vi "Save File DOE Configuration.vi"(5 "Add/Remove Enum":T1(ring)=enum."Update", 7 "Latest String Search":string[](array[string])=["TR Number:", "T0007456"], 8 "error in (no error)":errorcluster, 10 "File Save Configuration Data Path":path=path "C:/GE/Washer DOE/WasherDOEConfig.csv", 11 "Button Number":i32=16) -> (0 "error out":errorcluster, 2 "Updated List":string[](array[string]), 3 "Full Data Output":string[][](array[string])=[["Cycle Selection", "File Paths", "Laurel Meter IP (Cold/Hot)", "Agilent IP", "APLUS IP", "File Search", "ITHX Humidity Sensor IP Address", "Scale IP Address", "Agilent Channels (Analog)", "Agilent Channels (Temperature TC)", "", "Wash Temperature", "Rinse Temperature", "Load Size", "Model Detail Header", "EOC Commands", "Manufacturer-Dish", "Unit Control-Dish", "Test Type:", "Cycle Mode-Dish", "Inlet Temperature-Dish", "Detergent-Dish", "Washer Header Detail", "Dishwasher Header Detail", "TC1 Coefficients (A_B_C)", "TC2 Coefficients (A_B_C)", "TC3 Coefficients (A_B_C)", "TC4 Coefficients (A_B_C)", "TC5 Coefficients (A_B_C)", "TC6 Coefficients (A_B_C)", "TC7 Coefficients (A_B_C)", "TR Number:", "Lab ID:", "Station ID:", "Technician:", "Water Pressure (PSI):", "Ambient RH:", "Supply Voltage:", "Frequency:", "Build:", "Hot Water Temperature (Fahrenheit)", "Cold Water Temperature (Fahrenheit)", "Heating Mode"], ["Eco Wash", "C:\\GE\\Washer DOE\\CalibrationDates.txt", "10.0.3.67", "169.254.9.72", "10.0.3.101", "DOE Template", "10.0.3.139", "10.0.3.5", "101", "111", "", "Extra Hot", "Cold", "Max", "TR Number:", "EOC", "GE", "Electronic", "Kitchen", "Auto", "110", "Cascade", "Program Name:", "Manufacturer:", "0", "0", "0", "0", "0", "0", "0", "", "", "Station 1", "Test", "25", "50", "110", "50", "DG", "120", "50", "Heat Pump"], ["Standard Wash", "C:\\GE\\Washer DOE\\DOE Capacity.txt", "10.0.3.66", "", "", "Rev", "", "", "102", "112", "", "Hot", "Hot Rinse", "Min", "Lab ID:", "ShuttingDown", "Electrolux", "Mechanical", "DOE", "Pots & Pans", "120", "Dawn", "Model Family:", "Unit Control:", "0", "0", "0", "0", "0", "0", "0", "", "", "Station 2", "", "30", "60", "115", "60", "DC", "130", "58", "Hybrid"], ["Heavy Wash", "C:\\GE\\Washer DOE", "", "", "", "xltm", "", "", "113", "", "", "Warm 1", "", "Avg", "Test Name:", "", "Mabe", "", "Portable Test", "Quick", "130", "Gain", "Cycle Selection:", "Test Type:", "0", "0", "0", "0", "0", "0", "0", "", "", "Station 3", "", "35", "80", "120", "80", "Pre-Pilot", "135", "68", "Boost"], ["test", "\\\\3.67.38.12\\share\\Test Data\\Washer DOE\\Models", "", "", "", "", "", "", "114", "", "", "Warm 2", "", "Max1*", "Model:", "", "Bosch", "", "", "", "135", "", "Wash Temperature:", "Cycle Mode:", "", "", "", "", "", "", "", "", "", "Station 4", "", "40", "60", "140", "", "Production", "140", "", "Standard"], ["", "D:\\data\\WasherDOE", "", "", "", "", "", "", "115", "", "", "Warm 3", "", "Max2**", "Serial Number:", "", "Whirlpool", "", "", "", "140", "", "Rinse Temperature:", "Inlet Temperature (F):", "", "", "", "", "", "", "", "", "", "Station 5", "", "", "", "", "", "", "", "", "Vacation"], ["", "C:\\GE\\Washer DOE\\DOE_Backup.ini", "", "", "", "", "", "", "116", "", "", "Cold", "", "", "Station ID:", "", "", "", "", "", "", "", "Load Size:", "Detergent:", "", "", "", "", "", "", "", "", "", "Station 6", "", "", "", "", "", "", "", "", ""], ["", "", "", "", "", "", "", "", "", "", "", "Note", "", "", "Engineer:", "", "", "", "", "", "", "", "Hot Water Temperature (Fahrenheit):", "Auto Cup Weight (gm):", "", "", "", "", "", "", "", "", "", "Station 7", "", "", "", "", "", "", "", "", ""], ["", "", "", "", "", "", "", "", "", "", "", "", "", "", "Technician", "", "", "", "", "", "", "", "Cold Water Temperature (Fahrenheit):", "Open Cup Weight (gm):", "", "", "", "", "", "", "", "", "", "Station 8", "", "", "", "", "", "", "", "", ""], ["", "", "", "", "", "", "", "", "", "", "", "", "", "", "Water Pressure:", "", "", "", "", "", "", "", "Capacity (cu.ft)", "", "", "", "", "", "", "", "", "", "", "Station 9", "", "", "", "", "", "", "", "", ""], ["", "", "", "", "", "", "", "", "", "", "", "", "", "", "Ambient RH:", "", "", "", "", "", "", "", "Initial Cloth Weight:", "", "", "", "", "", "", "", "", "", "", "Station 10", "", "", "", "", "", "", "", "", ""], ["", "", "", "", "", "", "", "", "", "", "", "", "", "", "Supply Voltage:", "", "", "", "", "", "", "", "Cloth Lot:", "", "", "", "", "", "", "", "", "", "", "Station 11", "", "", "", "", "", "", "", "", ""], ["", "", "", "", "", "", "", "", "", "", "", "", "", "", "Frequency:", "", "", "", "", "", "", "", "", "", "", "", "", "", "", "", "", "", "", "Station 12", "", "", "", "", "", "", "", "", ""], ["", "", "", "", "", "", "", "", "", "", "", "", "", "", "Build:", "", "", "", "", "", "", "", "", "", "", "", "", "", "", "", "", "", "", "", "", "", "", "", "", "", "", "", ""]])   [LabVIEW 2023, in "File Setup.lvlib"]
uses:
  File Setup.lvlib
  <vilib>/Utility/file.llb/Read Delimited Spreadsheet (string).vi
  <vilib>/Utility/file.llb/Write Delimited Spreadsheet (string).vi
panel:
  in  "Configuration Tab":enum32{"Main", "Default Data", "Configuration"}(tab)=enum."Default Data"
  in  "Calibration Data":string[][](array[string])
  in  "Update":bool
  out "Default Data Output":string[][](array[string])
  out "Coeffficient C":dbl
  out "Coeffficient B":dbl
  out "Coeffficient A":dbl
  in  "Get Coefficients":bool
  in  "TC Inputs":string[][](array[string])=[["Temperature Setpoint", "Sourced TC Temperature (F)", "Measured TC Temperature (F)"], ["1", "", ""], ["2", "", ""], ["3", "", ""]]
  in  "Debug Tab":enum32{"Input", "Output"}(tab)
  in  "Debug":bool=TRUE
  out "States":string[](array[string])=["Macro: Initialize", "Data: Initialize", "Initialize Core Data", "UI: Initialize", "UI: Front Panel State", "Read Current Data"]
  # "Configuration File Update"
  # "Calculate TC Coefficients"
  # "Agilent Syntax\n\nY=Gain*x+Offset = (Gain_Offset_Name)Channel_AG# or (5.23_3.4_TC1)107_1"
  # "Kitchen TC Layout\n\n1) TC Jack 1\n2) TC Jack 2\n3) TC Jack 3\n4) TC Jack 4\n5) TC Jack 5\n6) TC Jack 6\n7) Hot Water TC"
  # "Washer DOE\n\n1) TC1 Cold Water Temp\n2) TC2 Hot Water Temp\n3) N/A\n4) N/A\n5) N/A\n6) N/A\n7) N/A"
  # "Portable Adv Sys\n\n1) TC1 Cold Water Temp\n2) TC2 Hot Water Temp\n3) N/A\n4) N/A\n5) N/A\n6) N/A\n7) N/A"
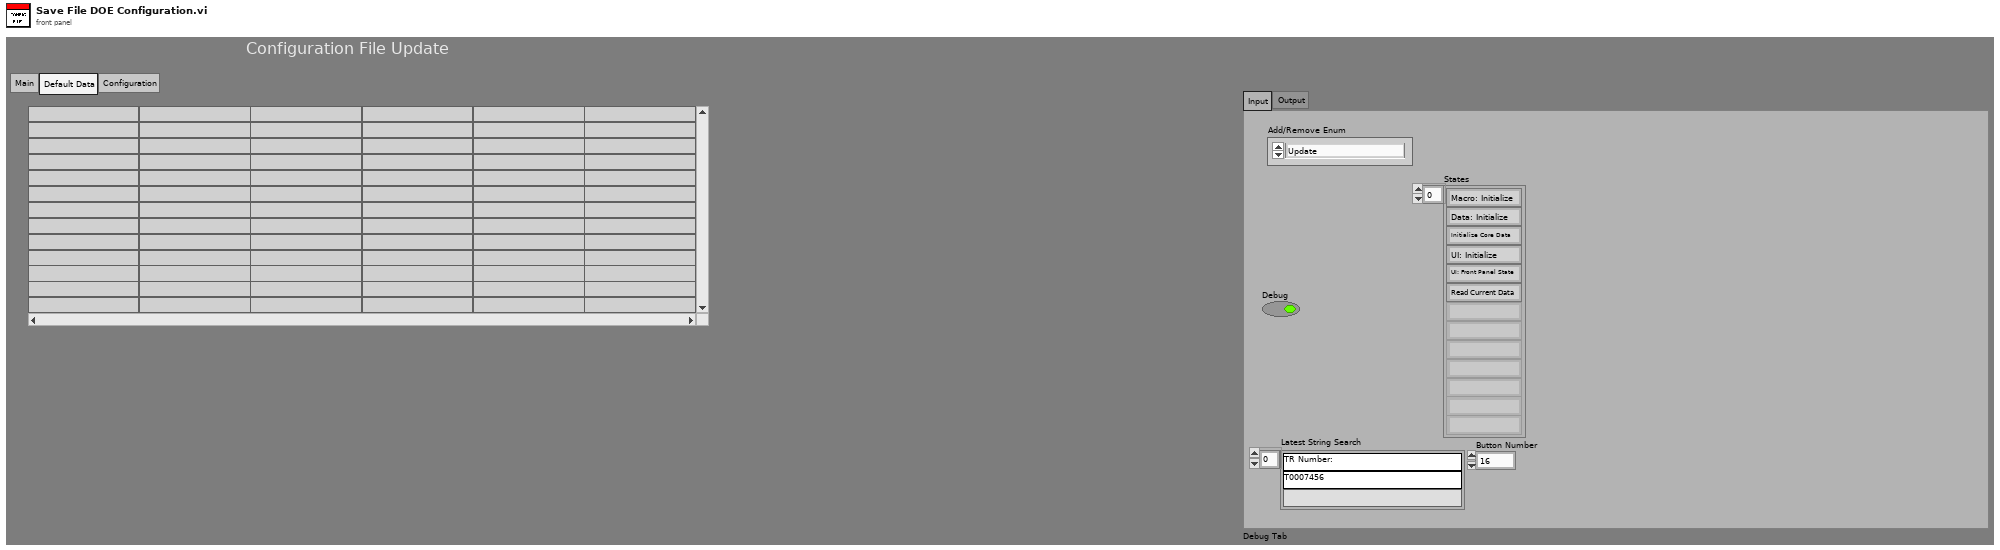
[diagram p1: front panel]
types:
  T1 = enum16{"Load Standard", "Remove", "Add", "Update"}
  T2 = enum32{"invalid app kind", "Development System", "Run Time System", "Student Edition", "Embedded LabVIEW", "Evaluation", "Custom"}
  T3 = enum32{"Invalid", "Standard", "Closed", "Hidden", "Minimized", "Maximized"}
  T4 = cluster{"Core":cluster{"Current VI Reference":refnum<vi>, "Close Panel on Exit?":bool}, "File Save Configuration Data Path":path, "Full Data":string[][], "Button Number":i32, "Latest String Search":string[], "Updated List":string[]}
  T5 = cluster{"Current VI Reference":refnum<vi>, "Close Panel on Exit?":bool}
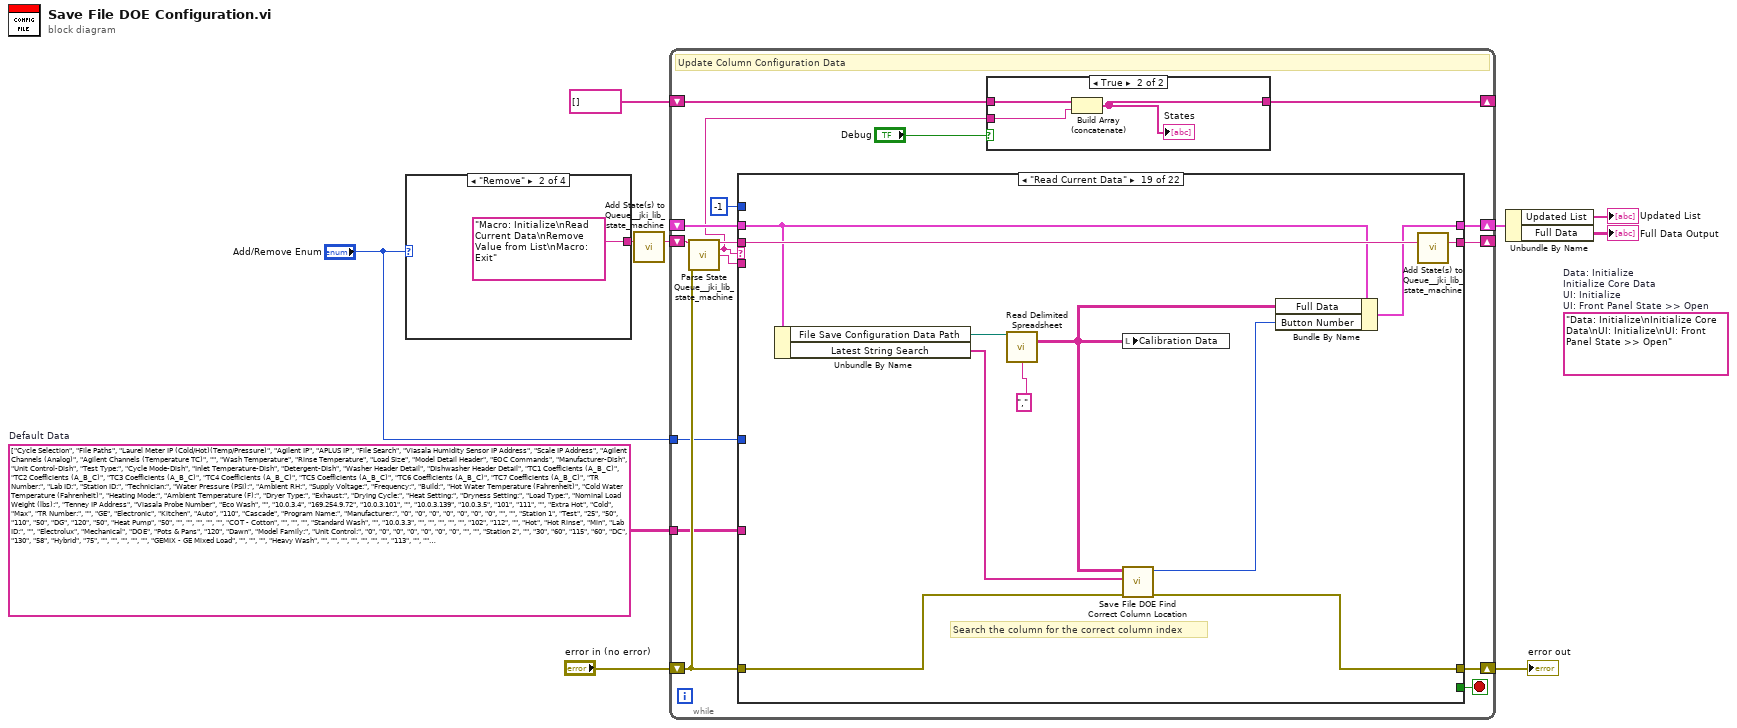
[diagram p0: block diagram]
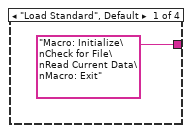
[diagram p2: hidden frame]
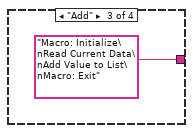
[diagram p3: hidden frame]
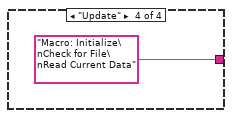
[diagram p4: hidden frame]
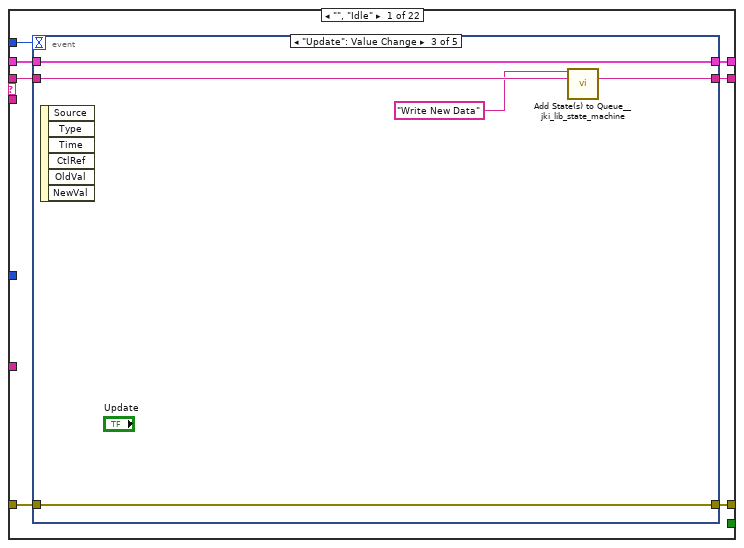
[diagram p6: hidden frame]
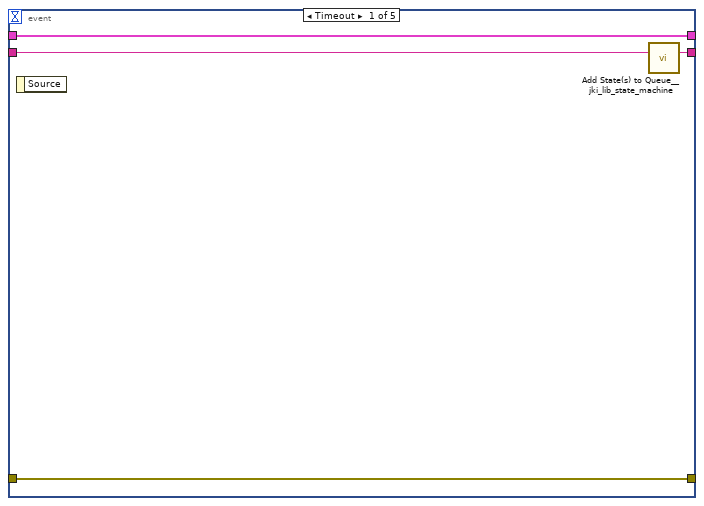
[diagram p7: hidden frame]
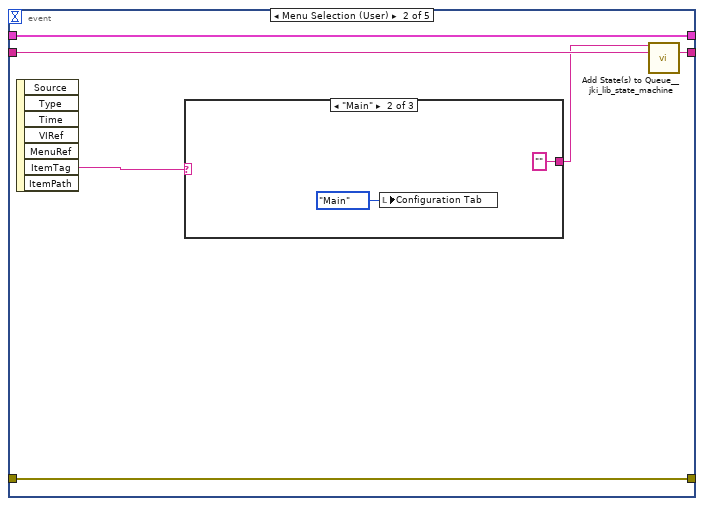
[diagram p8: hidden frame]
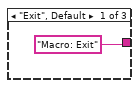
[diagram p9: hidden frame]
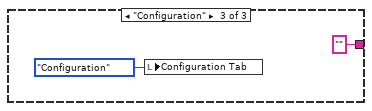
[diagram p10: hidden frame]
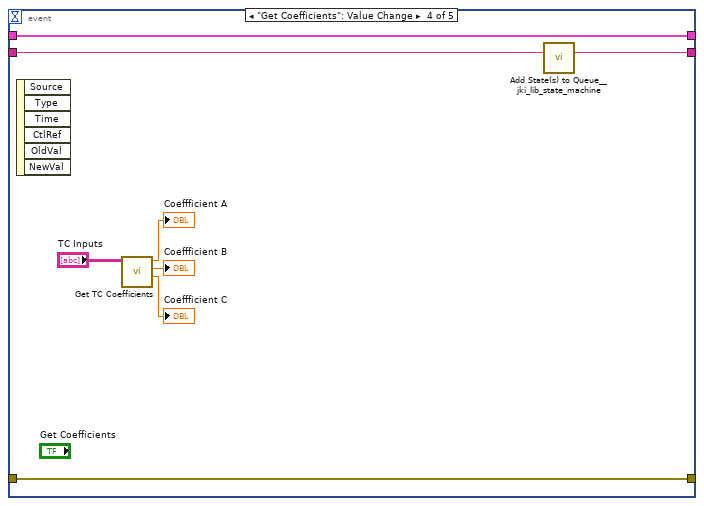
[diagram p11: hidden frame]
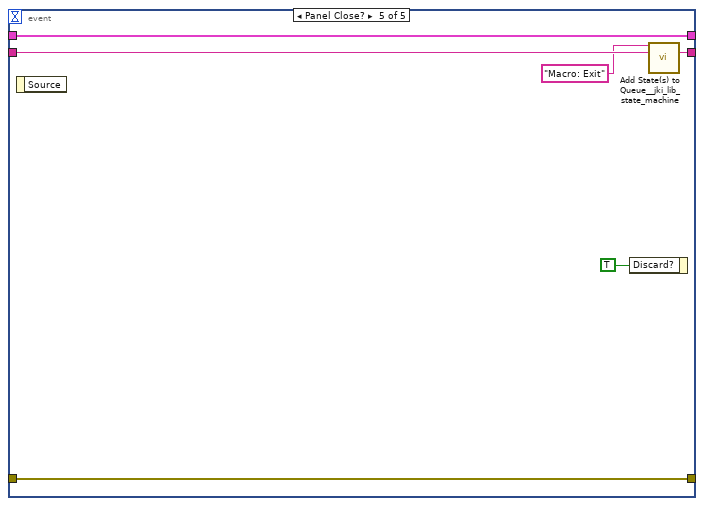
[diagram p12: hidden frame]
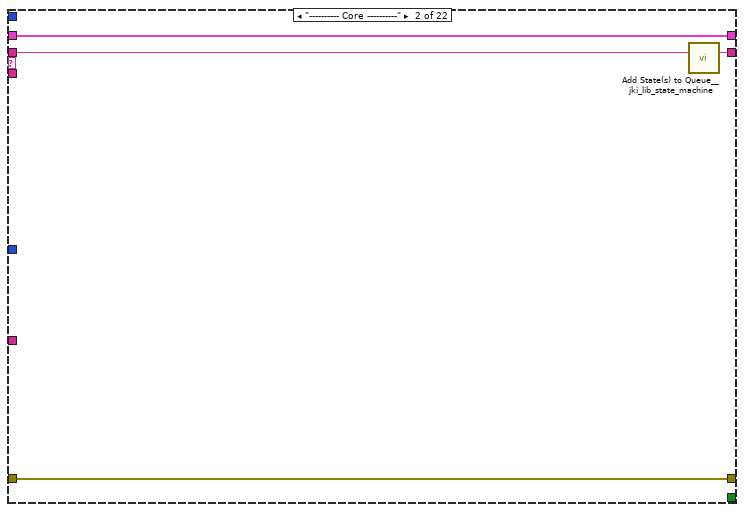
[diagram p13: hidden frame]
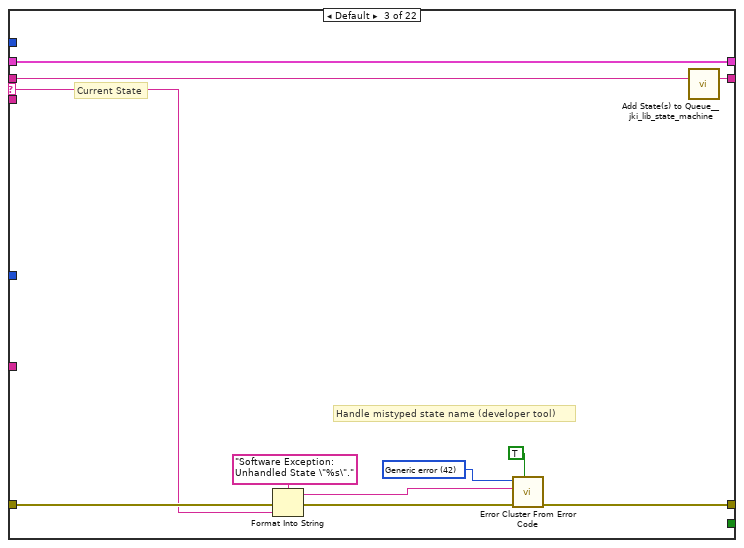
[diagram p14: hidden frame]
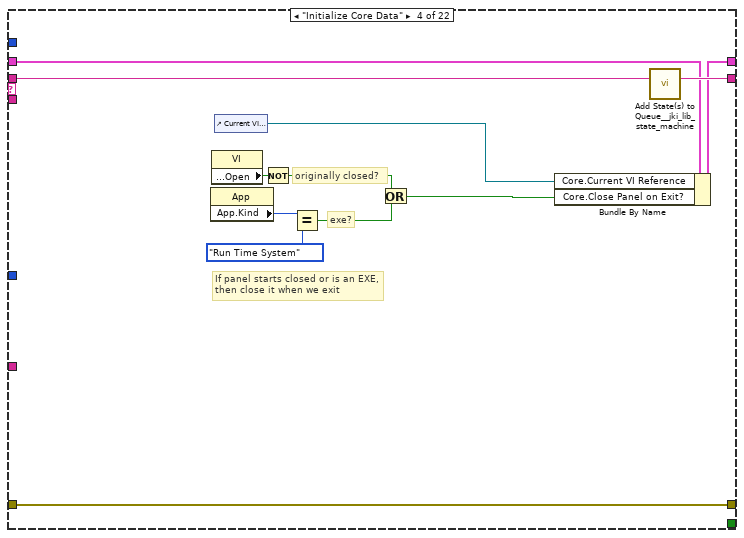
[diagram p15: hidden frame]
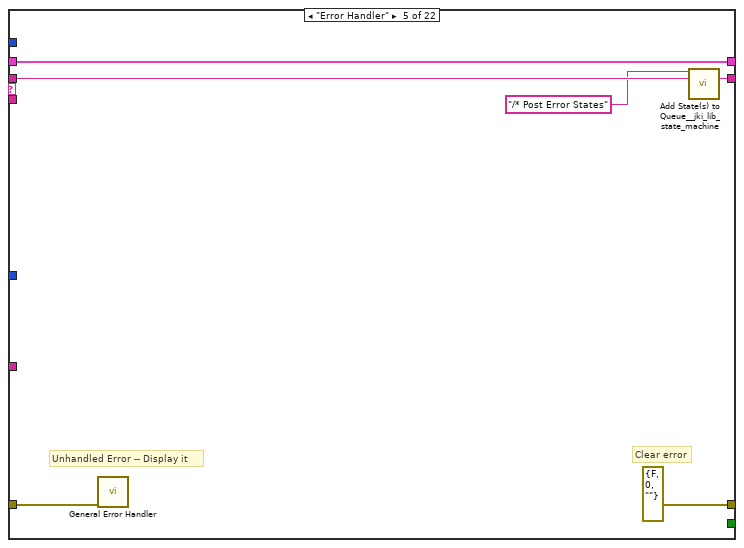
[diagram p16: hidden frame]
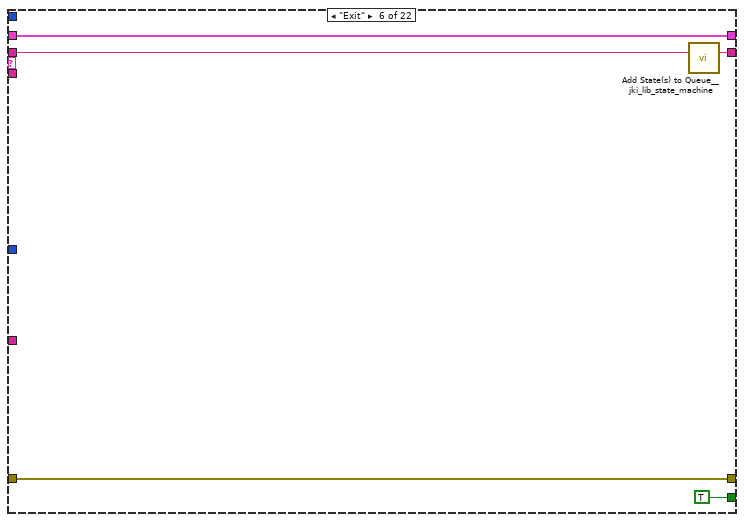
[diagram p17: hidden frame]
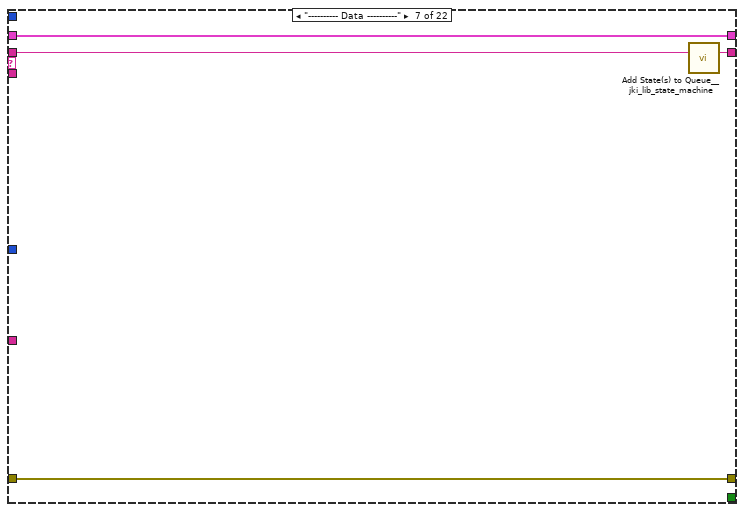
[diagram p18: hidden frame]
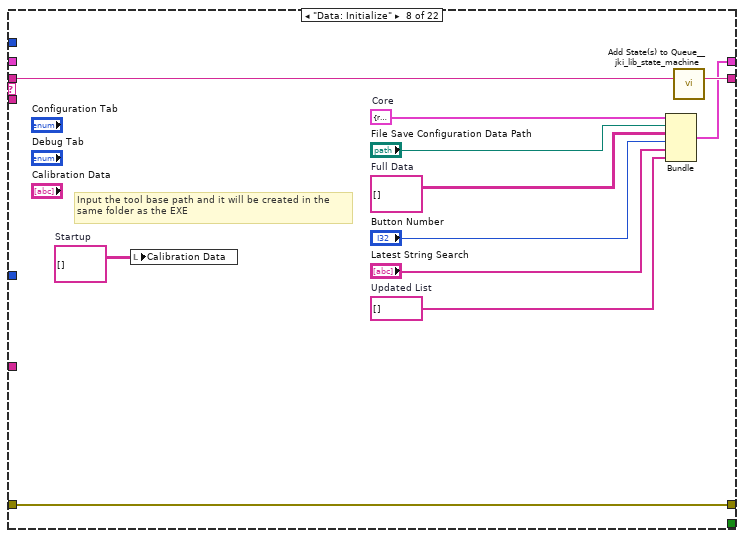
[diagram p19: hidden frame]
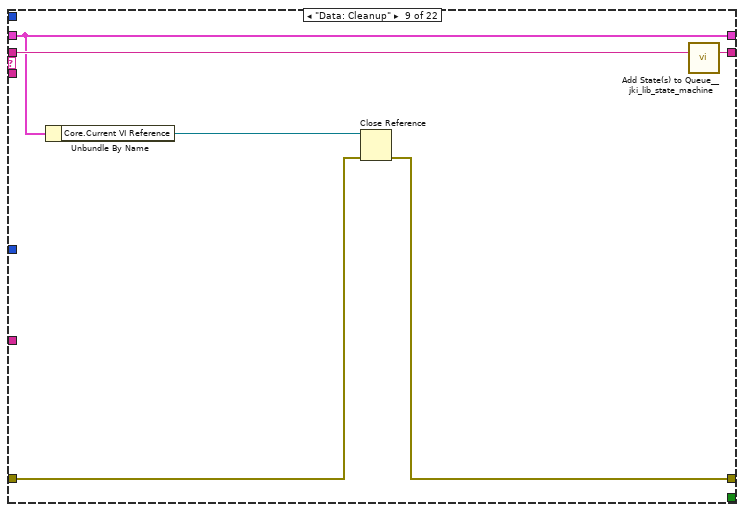
[diagram p20: hidden frame]
diagram:
  (unwired) "Data: Initialize\nInitialize Core Data\nUI: Initialize\nUI: Front Panel State >> Open"  # Data: Initialize Initialize Core Data UI: Initialize UI: Front Panel State >> Open
  w1 = string[][] [["Cycle Selection", "File Paths", "Laurel Meter IP (Cold/Hot)(Temp/Pressure)", "Agilent IP", "APLUS IP", "File Search", "Viasala Humidity Sensor IP Address", "Scale IP Address", "Agilent Channels (Analog)", "Agilent Channels (Temperature TC)", "", "Wash Temperature", "Rinse Temperature", "Load Size", "Model Detail Header", "EOC Commands", "Manufacturer-Dish", "Unit Control-Dish", "Test Type:", "Cycle Mode-Dish", "Inlet Temperature-Dish", "Detergent-Dish", "Washer Header Detail", "Dishwasher Header Detail", "TC1 Coefficients (A_B_C)", "TC2 Coefficients (A_B_C)", "TC3 Coefficients (A_B_C)", "TC4 Coefficients (A_B_C)", "TC5 Coefficients (A_B_C)", "TC6 Coefficients (A_B_C)", "TC7 Coefficients (A_B_C)", "TR Number:", "Lab ID:", "Station ID:", "Technician:", "Water Pressure (PSI):", "Ambient RH:", "Supply Voltage:", "Frequency:", "Build:", "Hot Water Temperature (Fahrenheit)", "Cold Water Temperature (Fahrenheit)", "Heating Mode:", "Ambient Temperature (F):", "Dryer Type:", "Exhaust:", "Drying Cycle:", "Heat Setting:", "Dryness Setting:", "Load Type:", "Nominal Load Weight (lbs):", "Tenney IP Address", "Viasala Probe Number"], ["Eco Wash", "", "10.0.3.4", "169.254.9.72", "10.0.3.101", "", "10.0.3.139", "10.0.3.5", "101", "111", "", "Extra Hot", "Cold", "Max", "TR Number:", "", "GE", "Electronic", "Kitchen", "Auto", "110", "Cascade", "Program Name:", "Manufacturer:", "0", "0", "0", "0", "0", "0", "0", "", "", "Station 1", "Test", "25", "50", "110", "50", "DG", "120", "50", "Heat Pump", "50", "", "", "", "", "", "COT - Cotton", "", "", ""], ["Standard Wash", "", "10.0.3.3", "", "", "", "", "", "102", "112", "", "Hot", "Hot Rinse", "Min", "Lab ID:", "", "Electrolux", "Mechanical", "DOE", "Pots & Pans", "120", "Dawn", "Model Family:", "Unit Control:", "0", "0", "0", "0", "0", "0", "0", "", "", "Station 2", "", "30", "60", "115", "60", "DC", "130", "58", "Hybrid", "75", "", "", "", "", "", "GEMIX - GE Mixed Load", "", "", ""], ["Heavy Wash", "", "", "", "", "", "", "", "113", "", "", "Warm 1", "", "Avg", "Test Name:", "", "Mabe", "", "Portable Test", "Quick", "130", "Gain", "Cycle Selection:", "Test Type:", "0", "0", "0", "0", "0", "0", "0", "", "", "Station 3", "", "35", "80", "120", "80", "Pre-Pilot", "135", "68", "Boost", "90", "", "", "", "", "", "GEEZ - GE Easy Care", "", "", ""], ["test", "", "", "", "", "", "", "", "", "", "", "Warm 2", "", "Max1*", "Model:", "", "Bosch", "", "", "", "135", "", "Wash Temperature:", "Cycle Mode:", "", "", "", "", "", "", "", "", "", "Station 4", "", "40", "60", "140", "", "Production", "140", "", "Standard", "", "", "", "", "", "", "GEDEL - Ge Delicate Load (CU)", "", "", ""], ["", "C:\\data", "", "", "", "", "", "", "", "", "", "Warm 3", "", "Max2**", "Serial Number:", "", "Whirlpool", "", "", "", "140", "", "Rinse Temperature:", "Inlet Temperature (F):", "", "", "", "", "", "", "", "", "", "Station 5", "", "", "", "", "", "", "", "", "Vacation", "", "", "", "", "", "", "CU - CU Load", "", "", ""], ["", "C:\\GE\\Washer DOE\\DOE_Backup.ini", "", "", "", "", "", "", "", "", "", "Cold", "", "", "Station ID:", "", "", "", "", "", "", "", "Load Size:", "Detergent:", "", "", "", "", "", "", "", "", "", "Station 6", "", "", "", "", "", "", "", "", "", "", "", "", "", "", "", "DOE", "", "", ""], ["", "", "", "", "", "", "", "", "", "", "", "Note", "", "", "Engineer:", "", "", "", "", "", "", "", "Hot Water Temperature (Fahrenheit):", "Auto Cup Weight (gm):", "", "", "", "", "", "", "", "", "", "Station 7", "", "", "", "", "", "", "", "", "", "", "", "", "", "", "", "UL", "", "", ""], ["", "", "", "", "", "", "", "", "", "", "", "", "", "", "Technician", "", "", "", "", "", "", "", "Cold Water Temperature (Fahrenheit):", "Open Cup Weight (gm):", "", "", "", "", "", "", "", "", "", "Station 8", "", "", "", "", "", "", "", "", "", "", "", "", "", "", "", "AHAM", "", "", ""], ["", "", "", "", "", "", "", "", "", "", "", "", "", "", "Water Pressure:", "", "", "", "", "", "", "", "Capacity (cu.ft)", "", "", "", "", "", "", "", "", "", "", "Station 9", "", "", "", "", "", "", "", "", "", "", "", "", "", "", "", "GEACT", "", "", ""], ["", "", "", "", "", "", "", "", "", "", "", "", "", "", "Ambient RH:", "", "", "", "", "", "", "", "Initial Cloth Weight:", "", "", "", "", "", "", "", "", "", "", "Station 10", "", "", "", "", "", "", "", "", "", "", "", "", "", "", "", "", "", "", ""], ["", "", "", "", "", "", "", "", "", "", "", "", "", "", "Supply Voltage:", "", "", "", "", "", "", "", "Cloth Lot:", "", "", "", "", "", "", "", "", "", "", "Station 11", "", "", "", "", "", "", "", "", "", "", "", "", "", "", "", "", "", "", ""], ["", "", "", "", "", "", "", "", "", "", "", "", "", "", "Frequency:", "", "", "", "", "", "", "", "", "", "", "", "", "", "", "", "", "", "", "Station 12", "", "", "", "", "", "", "", "", "", "", "", "", "", "", "", "", "", "", ""], ["", "", "", "", "", "", "", "", "", "", "", "", "", "", "Build:", "", "", "", "", "", "", "", "", "", "", "", "", "", "", "", "", "", "", "", "", "", "", "", "", "", "", "", "", "", "", "", "", "", "", "", "", "", ""]]  # Default Data
  n1 = case shown="\"Remove\"" "Add/Remove Enum" {
    tunnel: ["Macro: Initialize\nCheck for File\nRead Current Data\nMacro: Exit" "Macro: Initialize\nRead Current Data\nRemove Value from List\nMacro: Exit" "Macro: Initialize\nRead Current Data\nAdd Value to List\nMacro: Exit" "Macro: Initialize\nCheck for File\nRead Current Data"] -> w9
    frame "Load Standard", Default {
    }
    frame "Remove" {
    }
    frame "Add" {
    }
    frame "Update" {
    }
  }
  n2 = call <vilib>:"Add State(s) to Queue__jki_lib_state_machine.vi"("State(s) in (\"\")"=w9) -> ("States Out"=w10:string)  [unwired: 14 in]
  n3 = while "Update Column Configuration Data" {
    shift-right: [w24] -> w5
    shift-left: _ -> [w23]
    shift-right: [w27] -> w8
    shift-left: "error in (no error)" -> [w21]
    shift-right: [w26] -> _
    shift-left: w10 -> [w28]
    tunnel: "Add/Remove Enum" -> [w20]
    shift-right: [w17] -> _
    shift-left: string[] [] -> [w18]
    tunnel: w1 -> [w15]
    stop <- w25 stop-if-true
    # "Update Column Configuration Data"
    n4 = call <vilib>:"Parse State Queue__jki_lib_state_machine.vi"("State Queue"=w28, "Error In (no error)"=w21) -> ("Remaining States"=w30:string, "Current State"=w19:string, "Arguments"=w29:string)  [unwired: 11 in]
    n5 = case shown="\"Read Current Data\"" w19 {
      selector: w19 -> [_ _ w80 _ _ _ _ _ _ _ _ _ _ _ _ _ _ _ _ _ _ _]
      tunnel: w30 -> [w41 w79 w84 w102 w108 w113 w117 w128 w134 w138 w142 w148 w159 w185 w190 w200 w204 w213 w229 w238 w257 w276]
      tunnel: w29 -> [_ _ _ _ _ _ _ _ _ _ _ w143 w153 _ _ _ _ _ _ _ _ _]
      tunnel: w23 -> [w39 w76 w82 w93 w105 w111 w114 _ w129 w135 w139 w146 w155 w182 w187 w197 w201 w211 w225 w234 w252 w272]
      tunnel: [w38 w77 w86 w99 errorcluster {"status"=FALSE, "code"=0, "source"=""} ("error out") w110 w115 w125 w130 w136 w140 w144 w156 w183 w188 w198 w202 w206 w221 w236 w255 w274] -> w27
      tunnel: w21 -> [w37 w77 w85 w99 w104 w110 w115 w125 w131 w136 w140 w145 w157 w183 w188 w198 w202 w209 w222 w236 w255 w274]
      tunnel: [w40 w78 w83 w101 w107 w112 w116 w127 w133 w137 w141 w147 w158 w184 w189 w199 w203 w212 w228 w237 w256 w275] -> w26
      tunnel: [_ _ _ _ _ TRUE _ _ _ _ _ _ _ _ _ _ _ _ _ _ _ _] -> w25
      tunnel: [w36 w76 w82 w100 w105 w111 w114 w126 w129 w135 w139 w146 w155 w182 w187 w197 w201 w211 w224 w234 w251 w271] -> w24
      tunnel: -1 ("Timeout") -> [w35 _ _ _ _ _ _ _ _ _ _ _ _ _ _ _ _ _ _ _ _ _]
      tunnel: w20 -> [_ _ _ _ _ _ _ _ _ _ _ _ _ _ _ _ _ _ _ w232 _ _]
      tunnel: w15 -> [_ _ _ _ _ _ _ _ _ _ _ _ _ _ _ _ _ w205 _ _ _ _]
      frame "", "Idle" {
        n6 = event shown="[2] \"Update\": Value Change" {
          selector: _ -> [_ _ _ _ _]
          dyn-events: _ -> [_ _ _ _ _]
          timeout: w35 -> [_ _ _ _ _]
          tunnel: w41 -> [w45 w51 w59 w67 w75]
          tunnel: [w44 w50 w58 w66 w74] -> w40
          tunnel: w39 -> [w42 w48 w61 w69 w72]
          tunnel: [w43 w49 w60 w68 w73] -> w38
          tunnel: w37 -> [w43 w49 w60 w68 w73]
          tunnel: [w42 w48 w61 w69 w72] -> w36
          event Timeout {
            n7 = event-data() -> ()  [unwired: 1 in, 1 out]
            n8 = call <vilib>:"Add State(s) to Queue__jki_lib_state_machine.vi"("State(s) in (\"\")"=w45) -> ("States Out"=w44:string)  [unwired: 14 in]
          }
          event Menu Selection (User) {
            n9 = event-data() -> ("ItemTag"=w47:string)  [unwired: 1 in, 6 out]
            n10 = case shown="\"Main\"" w47 {
              tunnel: ["Macro: Exit" "" ""] -> w46
              frame "Exit", Default {
              }
              frame "Main" {
                n11 = local write "Configuration Tab"(enum32{"Main", "Default Data", "Configuration"}."Main" ("Configuration Tab")) -> ()
              }
              frame "Configuration" {
                n12 = local write "Configuration Tab"(enum32{"Main", "Default Data", "Configuration"}."Configuration" ("Configuration Tab")) -> ()
              }
            }
            n13 = call <vilib>:"Add State(s) to Queue__jki_lib_state_machine.vi"("State(s) in Front (\"\")"=w46, "State(s) in (\"\")"=w51) -> ("States Out"=w50:string)  [unwired: 13 in]
          }
          event "Update": Value Change {
            n14 = event-data() -> ()  [unwired: 1 in, 6 out]
            n15 = call <vilib>:"Add State(s) to Queue__jki_lib_state_machine.vi"("State(s) in Front (\"\")"="Write New Data" ("State(s) in Front (\"\")"), "State(s) in (\"\")"=w59) -> ("States Out"=w58:string)  [unwired: 13 in]
          }
          event "Get Coefficients": Value Change {
            n16 = event-data() -> ()  [unwired: 1 in, 6 out]
            n17 = call "Get TC Coefficients.vi"("TC Inputs"="TC Inputs") -> ("C"=→"Coeffficient C":dbl, "B"=→"Coeffficient B":dbl, "A"=→"Coeffficient A":dbl)  [unwired: 8 in]
            n18 = call <vilib>:"Add State(s) to Queue__jki_lib_state_machine.vi"("State(s) in (\"\")"=w67) -> ("States Out"=w66:string)  [unwired: 14 in]
          }
          event Panel Close? {
            n19 = event-data() -> ()  [unwired: 1 in, 1 out]
            n20 = event-data("Discard?"=TRUE) -> ()  [unwired: 1 in, 1 out]
            n21 = call <vilib>:"Add State(s) to Queue__jki_lib_state_machine.vi"("State(s) in Front (\"\")"="Macro: Exit", "State(s) in (\"\")"=w75) -> ("States Out"=w74:string)  [unwired: 13 in]
          }
        }
      }
      frame "---------- Core ----------" {
        n22 = call <vilib>:"Add State(s) to Queue__jki_lib_state_machine.vi"("State(s) in (\"\")"=w79) -> ("States Out"=w78:string)  [unwired: 14 in]
      }
      frame Default {
        w89 = 42 items=["No error", "Argument error", "Memory is full", "Out of zone", "End of file", "File already open", "Generic file I/O error", "File not found", "File permission error", "Disk is full", "Duplicate path", "Too many files open", "System feature not enabled", "Resource file not found", "Cannot add resource", "Resource not found", "Image not found", "Image memory error", "Pen does not exist", "Config type invalid", "Config token not found", "Config parse error", "Config memory error", "Bad external code format", "Bad external code offset", "External code not present", "Null window", "Destroy window error", "Null menu", "Print aborted", "Bad print record", "Print driver error", "Windows error during printing", "Memory error during printing", "Print dialog error", "Generic print error", "Invalid device refnum", "Device not found", "Device parameter error", "Device unit error", "Cannot open device", "Device call aborted", "Generic error", "Cancelled by user", "Object ID too low", "Object ID too high", "Object not in heap", "Unknown heap", "Unknown object (invalid DefProc)", "Unknown object (DefProc not in table)", "Message out of range", "Invalid (null) method", "Unknown message", "Manager call not supported", "Bad address", "Network operation in progress", "Network operation timed out", "Connection is busy", "Network attribute not supported", "Network error", "Address in use", "System out of memory", "Connection aborted", "Connection refused", "Not connected", "Already connected", "Connection closed", "Initialization error (interapplication manager)", "Bad occurrence", "Wait on unbound occurrence handler", "Occurrence queue overflow", "Datalog type conflict", "Unused", "Unrecognized type (interapplication manager)", "Memory corrupt", "Failed to make temporary DLL", "Old CIN version", "Drag socket not found", "Failed to load drop-object", "Failed to register OLE object", "Failed to release OLE object", "Format specifier type mismatch", "Unknown format specifier", "Too few format specifiers", "Too many format specifiers", "Scan failed", "Newer CIN version", "Error converting to variant", "Runtime menu error", "Password tampered", "Variant attribute not found", "Incompatible variant data type", "Event data is not available", "Event Store is not present", "Occurrence is not found", "Event Queue is not created", "Event info is not available", "Refnum passed is NULL", "Error retrieving Class GUID", "Error retrieving CoClass GUID", "Error retrieving TypeLib GUID.", "Bad built application magic bytes.", "Specific driver is different from the specific driver associated with the Logical Name.", "There is no session opened to the class driver.", "Max Error", "MAX - Error with config objects", "MAX - Error loading configuration", "MAX - Group not supported"]
        # "Current State"
        # "Handle mistyped state name (developer tool)"
        n23 = Format Into String(format string="Software Exception: Unhandled State \"%s\"." ("message"), error in=w85, w80) -> (resulting string=w88:string, error out=w87:errorcluster)  [unwired: 1 in]
        n24 = call <vilib>:"Error Cluster From Error Code.vi"("show call chain? (False)"=TRUE, "error in (no error)"=w87, "error message (\"\")"=w88, "error code (0)"=w89) -> ("error out"=w86:errorcluster)  [unwired: 5 in]
        n25 = call <vilib>:"Add State(s) to Queue__jki_lib_state_machine.vi"("State(s) in (\"\")"=w84) -> ("States Out"=w83:string)  [unwired: 14 in]
      }
      frame "Initialize Core Data" {
        # "originally closed?"
        # "exe?"
        # "If panel starts closed or is an EXE, then close it when we exit"
        n26 = property class="App"() -> ("App.Kind"=w97:T2)  [unwired: 2 in, 2 out]
        n27 = property class="VI"() -> ("Front Panel.Open"=w98:bool)  [unwired: 2 in, 2 out]
        n28 = control-ref of="Current VI Reference"() -> (w91:refnum<vi>)
        n29 = Not(x=w98) -> (.not. x?=w95:bool)
        n30 = Equal?(x=w97, y=T2."Run Time System" ("Application:Kind")) -> (x = y?=w94:bool)
        n31 = Or(x=w95, y=w94) -> (x .or. y?=w92:bool)
        n32 = Bundle By Name(cluster=w93, "Core.Current VI Reference"=w91, "Core.Close Panel on Exit?"=w92) -> (w100:T4)
        n33 = call <vilib>:"Add State(s) to Queue__jki_lib_state_machine.vi"("State(s) in (\"\")"=w102) -> ("States Out"=w101:string)  [unwired: 14 in]
      }
      frame "Error Handler" {
        # "Unhandled Error -- Display it"
        # "Clear error"
        n34 = call <vilib>:"General Error Handler.vi"("error in (no error)"=w104) -> ()  [unwired: 10 in, 5 out]
        n35 = call <vilib>:"Add State(s) to Queue__jki_lib_state_machine.vi"("State(s) in Front (\"\")"="/* Post Error States", "State(s) in (\"\")"=w108) -> ("States Out"=w107:string)  [unwired: 13 in]
      }
      frame "Exit" {
        n36 = call <vilib>:"Add State(s) to Queue__jki_lib_state_machine.vi"("State(s) in (\"\")"=w113) -> ("States Out"=w112:string)  [unwired: 14 in]
      }
      frame "---------- Data ----------" {
        n37 = call <vilib>:"Add State(s) to Queue__jki_lib_state_machine.vi"("State(s) in (\"\")"=w117) -> ("States Out"=w116:string)  [unwired: 14 in]
      }
      frame "Data: Initialize" {
        w119 = string[][] []  # Startup
        w121 = string[] []  # Updated List
        w123 = string[][] []  # Full Data
        w124 = T5 {"Current VI Reference"=refnum, "Close Panel on Exit?"=TRUE}  # Core
        # "Input the tool base path and it will be created in the \nsame folder as the EXE"
        n38 = local write "Calibration Data"(w119) -> ()
        n39 = Bundle("Core"=w124, "File Save Configuration Data Path"="File Save Configuration Data Path", "Full Data"=w123, "Button Number"="Button Number", "Latest String Search"="Latest String Search", "Updated List"=w121) -> (w126:T4)  [unwired: 1 in]
        n40 = call <vilib>:"Add State(s) to Queue__jki_lib_state_machine.vi"("State(s) in (\"\")"=w128) -> ("States Out"=w127:string)  [unwired: 14 in]
      }
      frame "Data: Cleanup" {
        n41 = Unbundle By Name(w129) -> ("Core.Current VI Reference"=w132:refnum<vi>)
        n42 = Close Reference(reference=w132, error in (no error)=w131) -> (error out=w130:errorcluster)
        n43 = call <vilib>:"Add State(s) to Queue__jki_lib_state_machine.vi"("State(s) in (\"\")"=w134) -> ("States Out"=w133:string)  [unwired: 14 in]
      }
      frame "---------- UI ----------" {
        n44 = call <vilib>:"Add State(s) to Queue__jki_lib_state_machine.vi"("State(s) in (\"\")"=w138) -> ("States Out"=w137:string)  [unwired: 14 in]
      }
      frame "UI: Initialize" {
        n45 = call <vilib>:"Add State(s) to Queue__jki_lib_state_machine.vi"("State(s) in (\"\")"=w142) -> ("States Out"=w141:string)  [unwired: 14 in]
      }
      frame "UI: Cursor Set" {
        # "Argument"
        n46 = case shown="\"Idle\", Default" w143 {
          tunnel: w145 -> [w150 w152]
          tunnel: [w149 w151] -> w144
          frame "Idle", Default {
            n47 = call <vilib>:"Unset Busy.vi"("error in (no error)"=w150) -> ("error out"=w149:errorcluster)  [unwired: 10 in]
          }
          frame "Busy" {
            n48 = call <vilib>:"Set Busy.vi"("error in (no error)"=w152) -> ("error out"=w151:errorcluster)  [unwired: 9 in, 1 out]
          }
        }
        n49 = call <vilib>:"Add State(s) to Queue__jki_lib_state_machine.vi"("State(s) in (\"\")"=w148) -> ("States Out"=w147:string)  [unwired: 14 in]
      }
      frame "UI: Front Panel State" {
        # "Argument"
        n50 = Unbundle By Name(w155) -> ("Core.Current VI Reference"=w154:refnum<vi>)
        n51 = case shown="\"Open\", Default" w153 {
          tunnel: w157 -> [w163 w176]
          tunnel: [w165 w177] -> w156
          tunnel: w154 -> [w164 w174]
          frame "Open", Default {
            n52 = property class="VI"(reference=w164, error in=w163) -> (reference out=w161:refnum<vi>, error out=w162:errorcluster, "Front Panel.Open"=w160:bool)
            n53 = case shown="False" w160 {
              tunnel: [w168 w171] -> w165
              tunnel: w162 -> [w167 w171]
              tunnel: w161 -> [w166 _]
              frame False {
                n54 = invoke class="VI" method="FP.Open"(reference=w166, error in=w167, "Activate"=TRUE, "State"=T3."Standard") -> (error out=w168:errorcluster)  [unwired: 1 in, 4 out]
              }
              frame True {
              }
            }
          }
          frame "Close" {
            n55 = property class="VI"(reference=w174, error in=w176) -> (reference out=w173:refnum<vi>, error out=w175:errorcluster, "Front Panel.Open"=w172:bool)
            n56 = case shown="True" w172 {
              tunnel: [w178 w181] -> w177
              tunnel: w175 -> [w178 w180]
              tunnel: w173 -> [_ w179]
              frame False {
              }
              frame True {
                n57 = invoke class="VI" method="FP.Close"(reference=w179, error in=w180) -> (error out=w181:errorcluster)  [unwired: 1 in, 2 out]
              }
            }
          }
        }
        n58 = call <vilib>:"Add State(s) to Queue__jki_lib_state_machine.vi"("State(s) in (\"\")"=w159) -> ("States Out"=w158:string)  [unwired: 14 in]
      }
      frame "---------- Macro ----------" {
        n59 = call <vilib>:"Add State(s) to Queue__jki_lib_state_machine.vi"("State(s) in (\"\")"=w185) -> ("States Out"=w184:string)  [unwired: 14 in]
      }
      frame "Macro: Initialize" {
        w186 = "Data: Initialize\nInitialize Core Data\nUI: Initialize\nUI: Front Panel State >> Open"  # Data: Initialize Initialize Core Data UI: Initialize UI: Front Panel State >> Open
        n60 = call <vilib>:"Add State(s) to Queue__jki_lib_state_machine.vi"("State(s) in Front (\"\")"=w186, "State(s) in (\"\")"=w190) -> ("States Out"=w189:string)  [unwired: 13 in]
      }
      frame "Macro: Exit" {
        n61 = Unbundle By Name(w197) -> ("Core.Close Panel on Exit?"=w196:bool)
        n62 = Select(t="UI: Front Panel State >> Close", s=w196, f="") -> (s? t:f=w193:string)
        n63 = call <vilib>:"Add State(s) to Queue__jki_lib_state_machine.vi"("State(s) in (\"\")"=w193, "State(s) at Back (\"\")"="Data: Cleanup\nExit") -> ("States Out"=w191:string)  [unwired: 13 in]
        n64 = call <vilib>:"Add State(s) to Queue__jki_lib_state_machine.vi"("State(s) in Front (\"\")"=w191, "State(s) in (\"\")"=w200) -> ("States Out"=w199:string)  [unwired: 13 in]
      }
      frame "---------- New Category ----------" {
        n65 = call <vilib>:"Add State(s) to Queue__jki_lib_state_machine.vi"("State(s) in (\"\")"=w204) -> ("States Out"=w203:string)  [unwired: 14 in]
      }
      frame "Check for File" {
        n66 = Unbundle By Name(w211) -> ("File Save Configuration Data Path"=w210:path)
        n67 = call <vilib>:"Check if File or Folder Exists.vi"("error in (no error)"=w209, "path"=w210) -> ("error out"=w207:errorcluster, "file or folder exists?"=w208:bool)  [unwired: 7 in, 1 out]
        n68 = case shown="True" w208 {
          tunnel: w205 -> [w217 _]
          tunnel: w210 -> [w216 _]
          tunnel: w207 -> [w215 w218]
          tunnel: [w214 w218] -> w206
          frame False {
            n69 = call "UTILITY Create Default File.vi"("Error In"=w215, "Default File"=w217, "Initial DOE Config"=w216) -> ("Error Out"=w214:errorcluster)  [unwired: 7 in, 1 out]
          }
          frame True {
          }
        }
        n70 = call <vilib>:"Add State(s) to Queue__jki_lib_state_machine.vi"("State(s) in (\"\")"=w213) -> ("States Out"=w212:string)  [unwired: 14 in]
        "Default Data Output" <- w205
      }
      frame "Read Current Data" {
        # "Search the column for the correct column index"
        n71 = Unbundle By Name(w225) -> ("File Save Configuration Data Path"=w227:path, "Latest String Search"=w220:string[])
        n72 = call-poly <vilib>:"Read Delimited Spreadsheet.vi"("file path (dialog if empty)"=w227, "delimiter (\\t)"="," ("delimiter (\\t)")) -> ("all rows"=w219:string[][])  [unwired: 8 in, 5 out]
        n73 = local write "Calibration Data"(w219) -> ()
        n74 = call "Save File DOE Find Correct Column Location.vi"("error in (no error)"=w222, "Search for Header"=w220, "Calibration With Header"=w219) -> ("error out"=w221:errorcluster, "Column Index Output"=w223:i32)  [unwired: 7 in]
        n75 = Bundle By Name(cluster=w225, "Full Data"=w219, "Button Number"=w223) -> (w224:T4)
        n76 = call <vilib>:"Add State(s) to Queue__jki_lib_state_machine.vi"("State(s) in (\"\")"=w229) -> ("States Out"=w228:string)  [unwired: 14 in]
      }
      frame "Write New Data" {
        # "If adding new functionality\nupdate. Used only in Debug Mode"
        n77 = Unbundle By Name(w234) -> ("File Save Configuration Data Path"=w233:path, "Full Data"=w231:string[][])
        n78 = case shown="\"Remove\", \"Add\"" w232 {
          tunnel: [w239 w240] -> w230
          tunnel: w231 -> [w239 _]
          frame "Remove", "Add" {
          }
          frame "Update", Default {
            n79 = local read "Calibration Data"() -> (w240:string[][])
          }
        }
        n80 = call-poly <vilib>:"Write Delimited Spreadsheet.vi"("file path (dialog if empty)"=w233, "2D data"=w230, "delimiter (\\t)"="," ("delimiter (\\t)")) -> ()  [unwired: 11 in, 2 out]
        n81 = call <vilib>:"Add State(s) to Queue__jki_lib_state_machine.vi"("State(s) in (\"\")"=w238) -> ("States Out"=w237:string)  [unwired: 14 in]
      }
      frame "Add Value to List" {
        # "Replace old dataset with new\ndataset"
        # "Strip off blank cells"
        n82 = Unbundle By Name(w252) -> ("Full Data"=w254:string[][], "Button Number"=w253:i32, "Latest String Search"=w245:string[])
        n83 = Index Array(array=w254, index (col)=w253) -> (element=w242:string[])  [unwired: 1 in]
        n84 = Index Array(array=w245, index=1) -> (element=w243:string)
        n85 = call "UTILITY Delete Empty String Cells.vi"("Array with Empty Cells"=w242) -> ("Array w/o Empty Cells"=w241:string[])  [unwired: 10 in]
        n86 = Build Array (concatenate)(w241, w243) -> (w248:string[])
        n87 = Replace Array Subset(array=w254, new element=w248, index (col)=w253) -> (w250:string[][])  [unwired: 1 in]
        n88 = Delete From Array(array=w248, index=0) -> (array with subset deleted=w246:string[])  [unwired: 1 in, 1 out]
        n89 = Bundle By Name(cluster=w252, "Full Data"=w250, "Updated List"=w246) -> (w251:T4)
        n90 = call <vilib>:"Add State(s) to Queue__jki_lib_state_machine.vi"("State(s) in Front (\"\")"="Write New Data" ("State(s) in Front (\"\")"), "State(s) in (\"\")"=w257) -> ("States Out"=w256:string)  [unwired: 13 in]
      }
      frame "Remove Value from List" {
        # "Update the controls\non the front panel"
        # "Strip off blank cells"
        n91 = Unbundle By Name(w272) -> ("Full Data"=w267:string[][], "Button Number"=w265:i32, "Latest String Search"=w262:string[])
        n92 = Index Array(array=w262, index=1) -> (element=w260:string)
        n93 = Index Array(array=w267, index (col)=w265) -> (element=w259:string[])  [unwired: 1 in]
        n94 = call "UTILITY Delete Empty String Cells.vi"("Array with Empty Cells"=w259) -> ("Array w/o Empty Cells"=w258:string[])  [unwired: 10 in]
        n95 = Delete From Array(array=w267, index (col)=w265) -> (array with subset deleted=w266:string[][])  [unwired: 2 in, 1 out]
        n96 = Search 1D Array(1D array=w258, element=w260) -> (index of element=w273:i32)  [unwired: 1 in]
        n97 = Delete From Array(array=w258, index=w273) -> (array with subset deleted=w264:string[])  [unwired: 1 in, 1 out]
        n98 = Delete From Array(array=w264, index=0) -> (array with subset deleted=w269:string[])  [unwired: 1 in, 1 out]
        n99 = Insert Into Array(array=w266, index (col)=w265, new element=w264) -> (w263:string[][])  [unwired: 1 in]
        n100 = Bundle By Name(cluster=w272, "Full Data"=w263, "Updated List"=w269) -> (w271:T4)
        n101 = call <vilib>:"Add State(s) to Queue__jki_lib_state_machine.vi"("State(s) in Front (\"\")"="Write New Data" ("State(s) in Front (\"\")"), "State(s) in (\"\")"=w276) -> ("States Out"=w275:string)  [unwired: 13 in]
      }
    }
    n102 = case shown="True" "Debug" {
      tunnel: w19 -> [_ w34]
      tunnel: w18 -> [w31 w33]
      tunnel: [w31 w32] -> w17
      frame False {
      }
      frame True {
        n103 = Build Array (concatenate)(w33, w34) -> (w32:string[])
        "States" <- w32
      }
    }
  }
  "error out" <- w8
  n104 = Unbundle By Name(w5) -> ("Updated List"=→"Updated List":string[], "Full Data"=→"Full Data Output":string[][])
